vi "XML - Get relative Configuration LLB_PPL path.vi"(10 "CD Template":refnum<class "NIVS_CD Template.lvclass">, 11 "Project Name":string) -> (3 "Relative Configuration LLB/PPL path":path)   [LabVIEW 2019, in "NIVS_Consolidated_CDW_MetaDataObj.lvclass"]
doc: "Create the relative path for the Configuration LLB based on the name and execution mode of the new custom device."
uses:
  NIVS_Consolidated_CDW_MetaDataObj.lvclass
  Template Classes/NIVS_CD Template/NIVS_CD Template.lvclass
  Build Spec System Explorer.ctl
  Build Spec System Explorer.vi
  Template Classes/NIVS_PPLCD Template/NIVS_PPLCD Template.lvclass
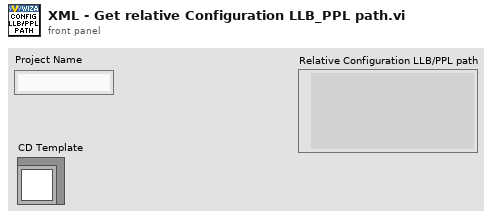
[diagram p1: front panel]
types:
  T1 = typedef "NIVS_Consolidated_CDW_MetaDataObj.lvclass/Build Spec System Explorer.ctl" = enum16{"Destinations.LLBFileName", "Destinations.PPLFileName"}
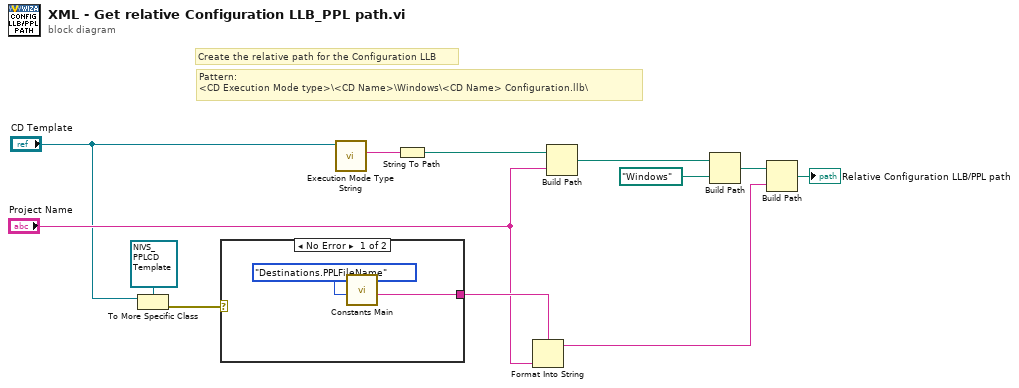
[diagram p0: block diagram]
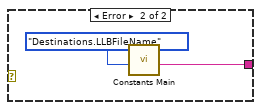
[diagram p2: hidden frame]
diagram:
  # "Create the relative path for the Configuration LLB"
  # "Pattern:\n<CD Execution Mode type>\\<CD Name>\\Windows\\<CD Name> Configuration.llb\\"
  n1 = To More Specific Class(target class=refnum<class "NIVS_PPLCD Template.lvclass"> refnum ("NIVS_PPLCD Template.lvclass"), reference="CD Template") -> (error out=w1:errorcluster)  [unwired: 1 in, 1 out]
  n2 = case shown="No Error" w1 {
    tunnel: [w13 w16] -> w10
    frame No Error {
      n3 = call-poly "Constants Main.vi"("Action"=Build_Spec_System_Explorer."Destinations.PPLFileName") -> ("Output"=w13:string)  [unwired: 10 in]
    }
    frame Error {
      n4 = call-poly "Constants Main.vi"("Action"=Build_Spec_System_Explorer."Destinations.LLBFileName") -> ("Output"=w16:string)  [unwired: 10 in]
    }
  }
  n5 = call-dynamic "Execution Mode Type String.vi"("CD Template"="CD Template") -> ("Execution Mode Type String"=w4:string)  [unwired: 10 in]
  n6 = String To Path(string=w4) -> (path=w9:path)
  n7 = Format Into String(format string=w10, "Project Name") -> (resulting string=w11:string)  [unwired: 2 in, 1 out]
  n8 = Build Path(base path=w9, name or relative path="Project Name") -> (appended path=w8:path)
  n9 = Build Path(base path=w8, name or relative path=path "Windows") -> (appended path=w6:path)
  n10 = Build Path(base path=w6, name or relative path=w11) -> (appended path=→"Relative Configuration LLB/PPL path":path)
